vi "NI_SAT_TEST_20150519_EXP.vi"() -> ()   [LabVIEW 2013]
panel:
  out "PXI1Slot4 3":dbl caption="Voltage Monitor Ouptute [1V/200V]" format="%.5f"
  out "Waveform Graph":dbl[](graph)
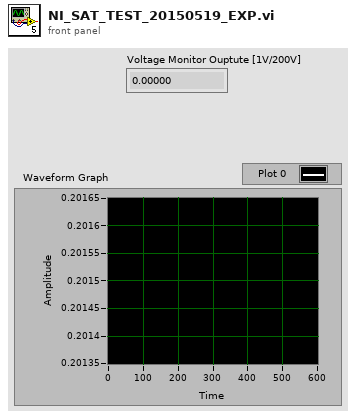
[diagram p1: front panel]
types:
  T1 = enum16{"open", "replace", "create", "open or create", "replace or create", "replace or create with confirmation"}
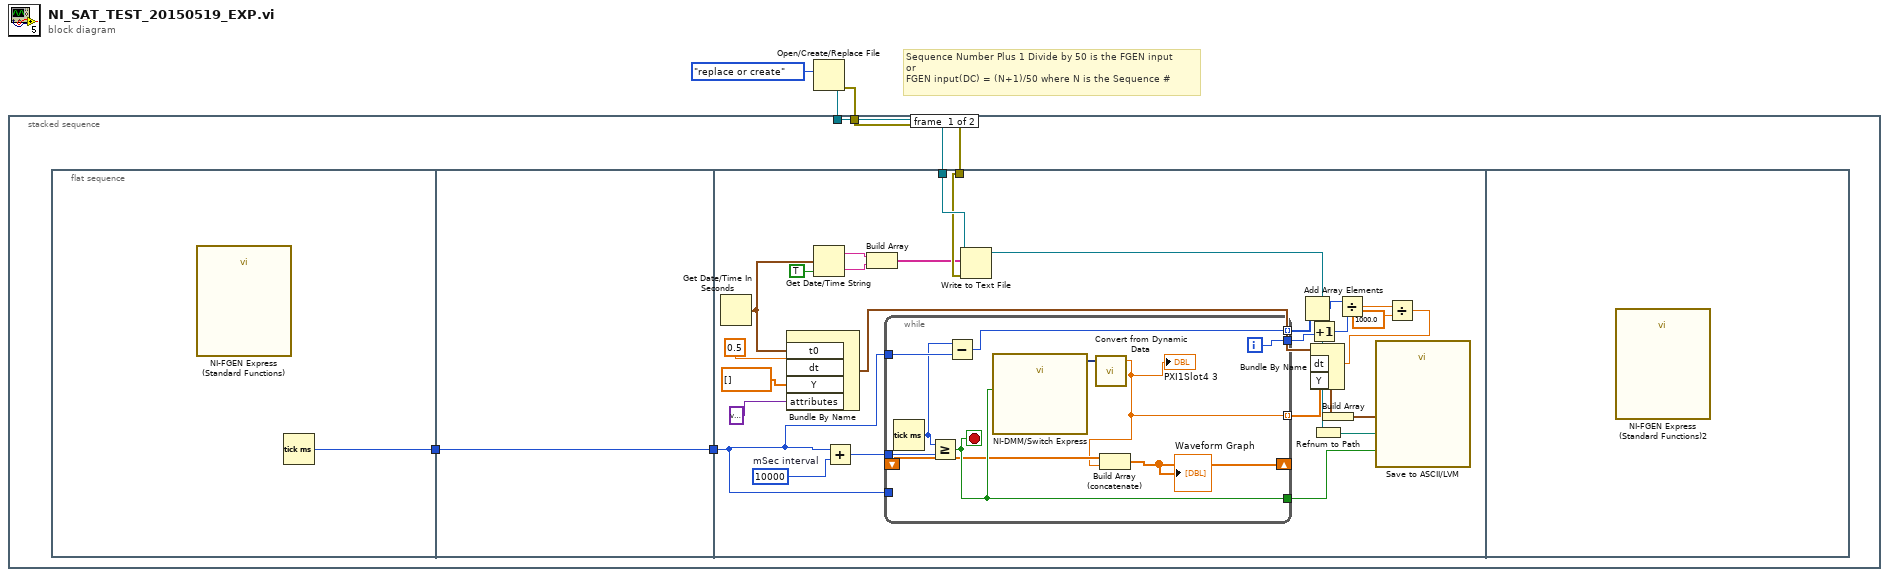
[diagram p0: block diagram]
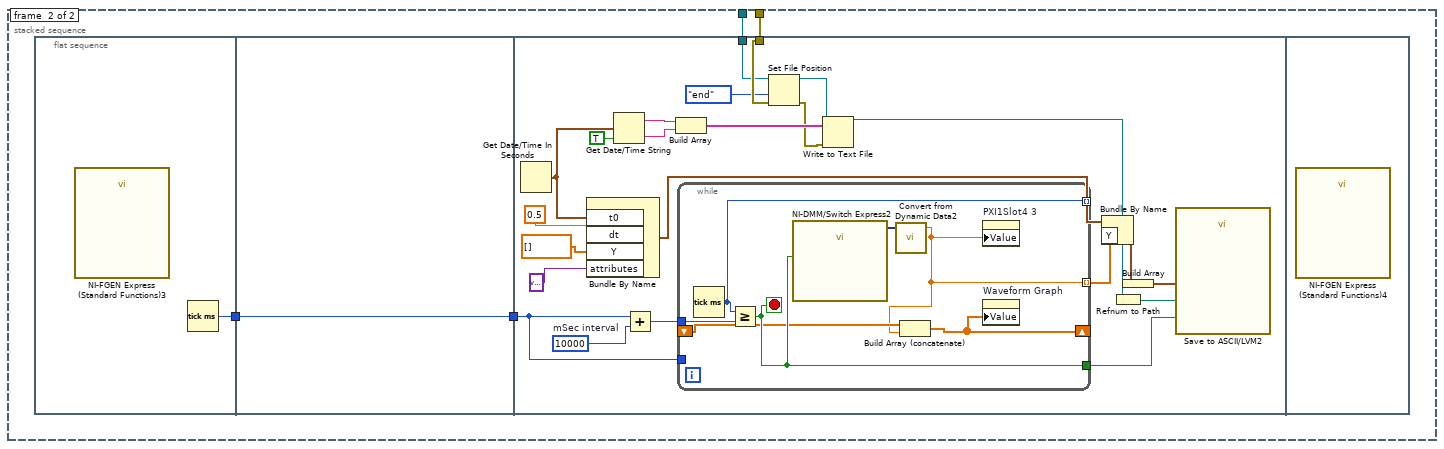
[diagram p2: hidden frame]
diagram:
  # "Sequence Number Plus 1 Divide by 50 is the FGEN input\nor\nFGEN input(DC) = (N+1)/50 where N is the Sequence #"
  n1 = Open/Create/Replace File(operation (0:open)=T1."replace or create") -> (refnum out=w3:refnum<file>, error out=w2:errorcluster)  [unwired: 5 in, 1 out]
  n2 = stacked-sequence {
    tunnel: w3 -> [w4 w48]
    tunnel: w2 -> [w5 w47]
    frame #0 {
      n3 = flat-sequence {
        tunnel: [w8] -> w7
        tunnel: w7 -> [w9]
        tunnel: [w9] -> w6
        tunnel: w6 -> [w19]
        tunnel: w4 -> [w26]
        tunnel: w5 -> [w25]
        frame #0 {
          n4 = call "NI-FGEN Express (Standard Functions)"() -> ()  [unwired: 11 in, 1 out]
          n5 = Tick Count (ms)() -> (millisecond timer value=w8:u32)
        }
        frame #1 {
        }
        frame #2 {
          w35 = u32 10000  # mSec interval
          n6 = Get Date/Time In Seconds() -> (seconds since 1Jan1904=w27:timestamp)
          n7 = Bundle By Name("t0"=w27, "dt"=0.5, "Y"=dbl[] [], "attributes"=variant) -> (w29:waveform(dbl))  [unwired: 1 in]
          n8 = Get Date/Time String(seconds (now)=w27, want seconds? (F)=TRUE) -> (date string=w24:string, time string=w23:string)  [unwired: 1 in]
          n9 = Add(x=w19, y=w35) -> (x+y=w36:u32)
          n10 = Build Array(w24, w23) -> (w22:string[])
          n11 = while "WhileLoop" {
            tunnel: w36 -> [w45]
            tunnel: [w44] -> w20
            tunnel: [w41] -> w30 mode=indexing
            tunnel: w19 -> [_]
            shift-right: [w42] -> _
            shift-left: _ -> [w43]
            tunnel: w19 -> [w40]
            tunnel: [w39] -> w18 mode=indexing
            tunnel: [w38] -> w15
            i -> [w38]
            stop <- w44 stop-if-true
            n12 = Tick Count (ms)() -> (millisecond timer value=w37:u32)
            n13 = Greater Or Equal?(x=w37, y=w45) -> (x >= y?=w44:bool)
            n14 = Subtract(x=w37, y=w40) -> (x-y=w39:u32)
            n15 = call "NI-DMM/Switch Express"("close (T)"=w44) -> ("signals out"=w46:dynamicdata)  [unwired: 16 in, 2 out]
            n16 = call "Convert from Dynamic Data"("Dynamic Data Type"=w46) -> ("Scalar"=w41:dbl)  [unwired: 3 in]
            "PXI1Slot4 3" <- w41
            n17 = Build Array (concatenate)(w43, w41) -> (w42:dbl[])
            "Waveform Graph" <- w42
          }
          n18 = Write to Text File(file (use dialog)=w26, text=w22, error in=w25) -> (refnum out=w21:refnum<file>)  [unwired: 1 in, 2 out]
          n19 = Add Array Elements(numeric array=w18) -> (sum=w17:u32)
          n20 = Increment(x=w15) -> (x+1=w16:i32)
          n21 = Refnum to Path(1:w21) -> (0:w11:path)
          n22 = Divide(x=w17, y=w16) -> (x/y=w14:dbl)
          n23 = Divide(x=w14, y=1000.0) -> (x/y=w12:dbl)
          n24 = Bundle By Name(cluster=w29, "dt"=w12, "Y"=w30) -> (w31:waveform(dbl))
          n25 = Build Array(w31) -> (w10:waveform(dbl)[])
          n26 = call "Save to ASCII/LVM"("signals in"=w10, "File Path"=w11, "close (T)"=w20) -> ()  [unwired: 16 in, 1 out]
        }
        frame #3 {
          n27 = call "NI-FGEN Express (Standard Functions)2"() -> ()  [unwired: 11 in, 1 out]
        }
      }
    }
    frame #1 {
      n28 = flat-sequence {
        tunnel: [w51] -> w50
        tunnel: w50 -> [w52]
        tunnel: [w52] -> w49
        tunnel: w49 -> [w70]
        tunnel: w48 -> [w55]
        tunnel: w47 -> [w58]
        frame #0 {
          n29 = call "NI-FGEN Express (Standard Functions)3"() -> ()  [unwired: 11 in, 1 out]
          n30 = Tick Count (ms)() -> (millisecond timer value=w51:u32)
        }
        frame #1 {
        }
        frame #2 {
          w74 = u32 10000  # mSec interval
          n31 = Get Date/Time In Seconds() -> (seconds since 1Jan1904=w64:timestamp)
          n32 = Bundle By Name("t0"=w64, "dt"=0.5, "Y"=dbl[] [], "attributes"=variant) -> (w66:waveform(dbl))  [unwired: 1 in]
          n33 = Get Date/Time String(seconds (now)=w64, want seconds? (F)=TRUE) -> (date string=w63:string, time string=w62:string)  [unwired: 1 in]
          n34 = Add(x=w70, y=w74) -> (x+y=w75:u32)
          n35 = Build Array(w63, w62) -> (w61:string[])
          n36 = while "WhileLoop" {
            tunnel: w75 -> [w81]
            tunnel: [w80] -> w53
            tunnel: [w77] -> w67 mode=indexing
            tunnel: w70 -> [_]
            shift-right: [w78] -> _
            shift-left: _ -> [w79]
            tunnel: [w76] -> _ mode=indexing
            stop <- w80 stop-if-true
            n37 = Tick Count (ms)() -> (millisecond timer value=w76:u32)
            n38 = Greater Or Equal?(x=w76, y=w81) -> (x >= y?=w80:bool)
            n39 = call "NI-DMM/Switch Express2"("close (T)"=w80) -> ("signals out"=w82:dynamicdata)  [unwired: 16 in, 2 out]
            n40 = call "Convert from Dynamic Data2"("Dynamic Data Type"=w82) -> ("Scalar"=w77:dbl)  [unwired: 3 in]
            n41 = Build Array (concatenate)(w79, w77) -> (w78:dbl[])
            n42 = property on="PXI1Slot4 3" class="DigNum (strict)"("Value"=w77) -> ()  [unwired: 2 in, 2 out]
            n43 = property on="Waveform Graph" class="WFGraph (strict)"("Value"=w78) -> ()  [unwired: 2 in, 2 out]
          }
          n44 = Set File Position(refnum=w55, from (0:start)=enum16{"start", "end", "current"}."end", error in=w58) -> (refnum out=w56:refnum<file>, error out=w57:errorcluster)  [unwired: 1 in]
          n45 = Write to Text File(file (use dialog)=w56, text=w61, error in=w57) -> (refnum out=w59:refnum<file>)  [unwired: 1 in, 2 out]
          n46 = Bundle By Name(cluster=w66, "Y"=w67) -> (w69:waveform(dbl))
          n47 = Refnum to Path(1:w59) -> (0:w60:path)
          n48 = Build Array(w69) -> (w68:waveform(dbl)[])
          n49 = call "Save to ASCII/LVM2"("signals in"=w68, "File Path"=w60, "close (T)"=w53) -> ()  [unwired: 16 in, 1 out]
        }
        frame #3 {
          n50 = call "NI-FGEN Express (Standard Functions)4"() -> ()  [unwired: 11 in, 1 out]
        }
      }
    }
  }
